vi "GetTxFrequency.vi"(6 "Legacy (f)?":bool, 8 "error in (no error)":errorcluster) -> (0 "error out":errorcluster, 2 "TxFreqs":dbl[](array[numeric]) format="%.2f")   [LabVIEW 2011]
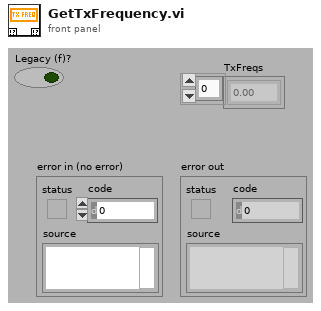
[diagram p1: front panel]
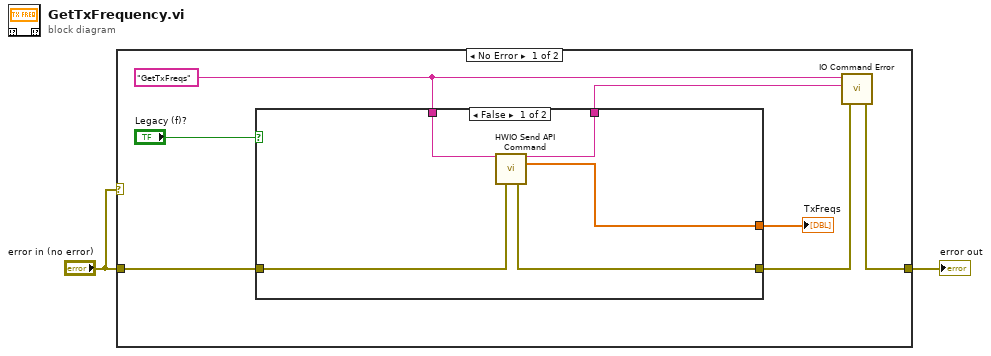
[diagram p0: block diagram]
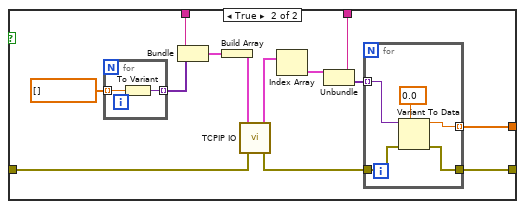
[diagram p2: hidden frame]
diagram:
  n1 = case shown="No Error" "error in (no error)" {
    tunnel: "error in (no error)" -> [w8 w35]
    tunnel: [w6 w35] -> w2
    frame No Error {
      w4 = "GetTxFreqs"
      n2 = case shown="False" "Legacy (f)?" {
        tunnel: [w12 w23] -> w9
        tunnel: w8 -> [w10 w22]
        tunnel: [w11 w20] -> w7
        tunnel: [w13 w19] -> w5
        tunnel: w4 -> [w14 w18]
        frame False {
          n3 = call "HWIO Send API Command.vi"("Action"=w14, "error in (no error)"=w10) -> ("Action out"=w13:string, "Double out"=w12:dbl[], "error out"=w11:errorcluster)  [unwired: 6 in, 5 out]
        }
        frame True {
          n4 = for {
            tunnel: [w34] -> w26 mode=indexing
            tunnel: dbl[] [] -> [w33] mode=indexing
            n5 = To Variant(anything=w33) -> (Variant=w34:variant)
          }
          n6 = Bundle(w18, w26) -> (w27:cluster{string, variant[]})  [unwired: 1 out]
          n7 = Build Array(w27) -> (w15:cluster{string, variant[]}[])
          n8 = call "TCPIP IO.vi"("error in (no error)"=w22, "Commands"=w15) -> ("error out"=w21:errorcluster, "Responses"=w17:cluster{string, variant[]}[])  [unwired: 1 in, 3 out]
          n9 = Index Array(array=w17) -> (element=w16:cluster{string, variant[]})  [unwired: 1 in]
          n10 = Unbundle(w16) -> (w19:string, w24:variant[])
          n11 = for {
            tunnel: [w32] -> w20
            tunnel: w21 -> [w31]
            tunnel: w24 -> [w29] mode=indexing
            tunnel: [w28] -> w23 mode=indexing
            n12 = Variant To Data(error in=w31, type=0.0, Variant=w29) -> (data=w28:dbl, error out=w32:errorcluster)
          }
        }
      }
      "TxFreqs" <- w9
      n13 = call "IO Command Error.vi"("error in (no error)"=w7, "Command Returned (\"\")"=w5, "Command Sent (\"\")"=w4) -> ("error out"=w6:errorcluster)  [unwired: 4 out]
    }
    frame Error {
    }
  }
  "error out" <- w2
